vi "Status Get Pressure Compensation.vi"(5 "Retry Attempts (0)":i32 min=0, 8 "error in":errorcluster, 11 "VISA resource name":refnum<visa-resource-name>) -> (0 "error out":errorcluster, 2 "User Compensation":i32, 3 "VISA resource name out":refnum<visa-resource-name>)   [LabVIEW 2020, in "ChromTech Series III Pump.lvlib"]
doc: "Returns the user flow rate compensation."
uses:
  <instrlib>/ChromTech Series III Pump/ChromTech Series III Pump.lvlib
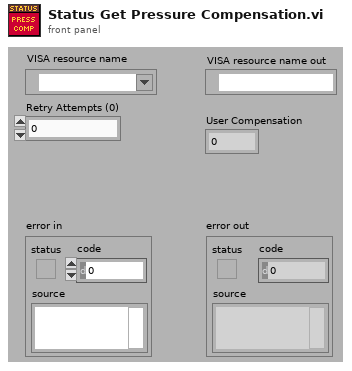
[diagram p1: front panel]
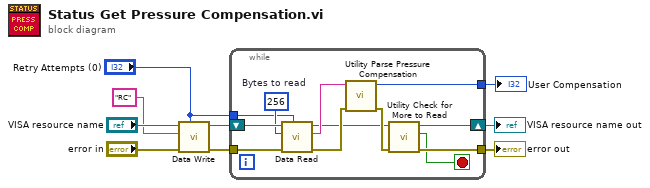
[diagram p0: block diagram]
diagram:
  n1 = call <instrlib>:"Data Write.vi"("Retry Attempts (0)"="Retry Attempts (0)", "error in (no error)"="error in", "Command"="RC", "VISA Refnum in"="VISA resource name") -> ("error out"=w5:errorcluster, "VISA Refnum out"=w4:refnum<visa-resource-name>)  [unwired: 6 in]
  n2 = while {
    tunnel: [w19] -> w6
    shift-right: [w12] -> w3
    shift-left: w4 -> [w17]
    tunnel: "Retry Attempts (0)" -> [w11]
    tunnel: w5 -> [w18]
    tunnel: [w14] -> w7
    stop <- w10 stop-if-true
    w16 = u32 256  # Bytes to read
    n3 = call <instrlib>:"Data Read.vi"("Retry Attempts (0)"=w11, "error in (no error)"=w18, "Bytes to read"=w16, "VISA Refnum in"=w17) -> ("error out"=w21:errorcluster, "read buffer"=w15:string, "VISA Refnum out"=w13:refnum<visa-resource-name>)  [unwired: 5 in]
    n4 = call <instrlib>:"Utility Parse Pressure Compensation.vi"("error in (no error)"=w21, "Input String"=w15) -> ("error out"=w20:errorcluster, "Compensation"=w19:i32)  [unwired: 8 in]
    n5 = call <instrlib>:"Utility Check for More to Read.vi"("error in (no error)"=w20, "VISA Refnum in"=w13) -> ("error out (unchanged)"=w14:errorcluster, "More to read?"=w10:bool, "VISA Refnum out"=w12:refnum<visa-resource-name>)  [unwired: 7 in]
  }
  "VISA resource name out" <- w3
  "error out" <- w7
  "User Compensation" <- w6
